vi "SALICRU_API_EMS.vi"() -> ()   [LabVIEW 2024]
panel:
  in  "stop":bool
  out "Values":map{string, dbl}(c390)
  out "Inverter alarms":i32[](array[numeric])
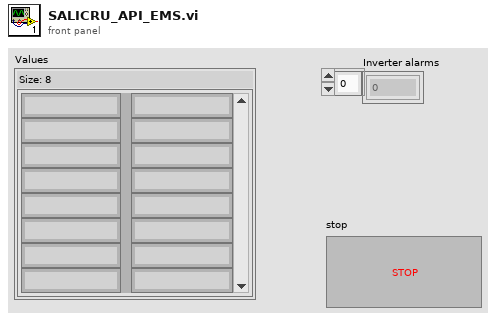
[diagram p1: front panel]
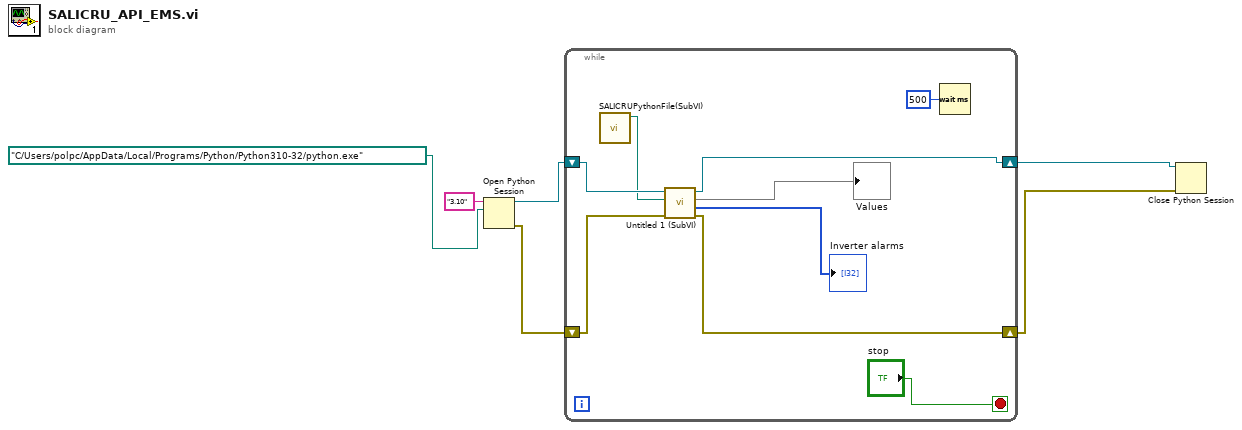
[diagram p0: block diagram]
diagram:
  n1 = Open Python Session(python version="3.10" ("Python version"), python path=path "C:/Users/polpc/AppData/Local/Programs/Python/Python310-32/python.exe") -> (session out=w3:refnum<k35>, error out=w4:errorcluster)  [unwired: 1 in]
  n2 = while {
    shift-right: [w13] -> w2
    shift-left: w3 -> [w11]
    shift-right: [w12] -> w1
    shift-left: w4 -> [w10]
    stop <- "stop" stop-if-true
    n3 = call "SALICRUPythonFile(SubVI).vi"() -> ("SALICRU WRAPPER FILE"=w9:path)  [unwired: 11 in]
    n4 = call "Untitled 1 (SubVI).vi"("error in (no error)"=w10, "Python File"=w9, "session in"=w11) -> ("error out"=w12:errorcluster, "Array"=→"Inverter alarms":i32[], "Map"=→"Values":map{string, dbl}, "session out"=w13:refnum<k35>)  [unwired: 5 in]
    n5 = Wait (ms)(milliseconds to wait=u32 500) -> ()  [unwired: 1 out]
  }
  n6 = Close Python Session(session in=w2, error in=w1) -> ()  [unwired: 1 out]
